vi "Escribir_Arreglo.vi"() -> ()   [LabVIEW 2016]
panel:
  in  "Stop Button":bool
  out "element":i32
  in  "disabled index (col)":i32
  in  "index (row)":i32
  out "Array":i32[][](array[numeric])
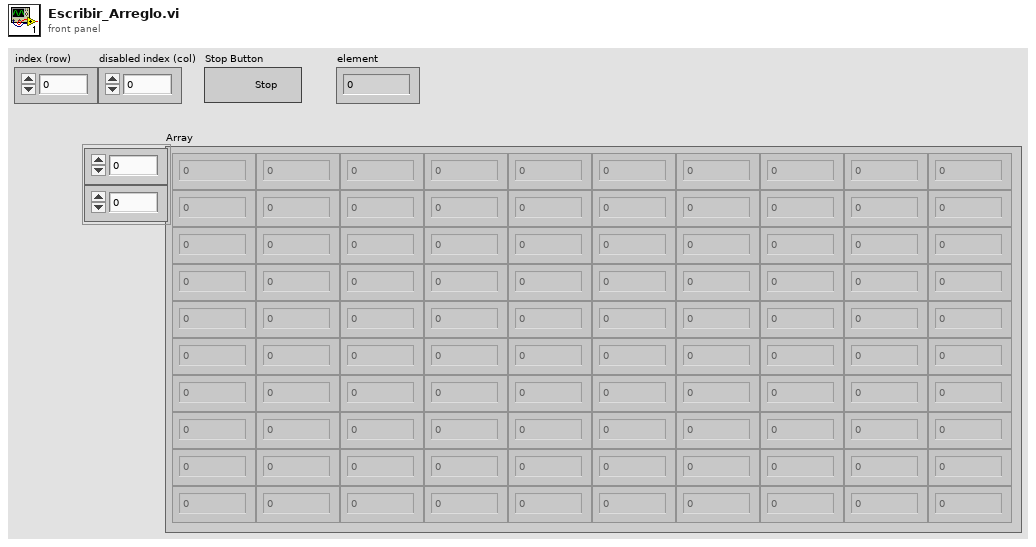
[diagram p1: front panel]
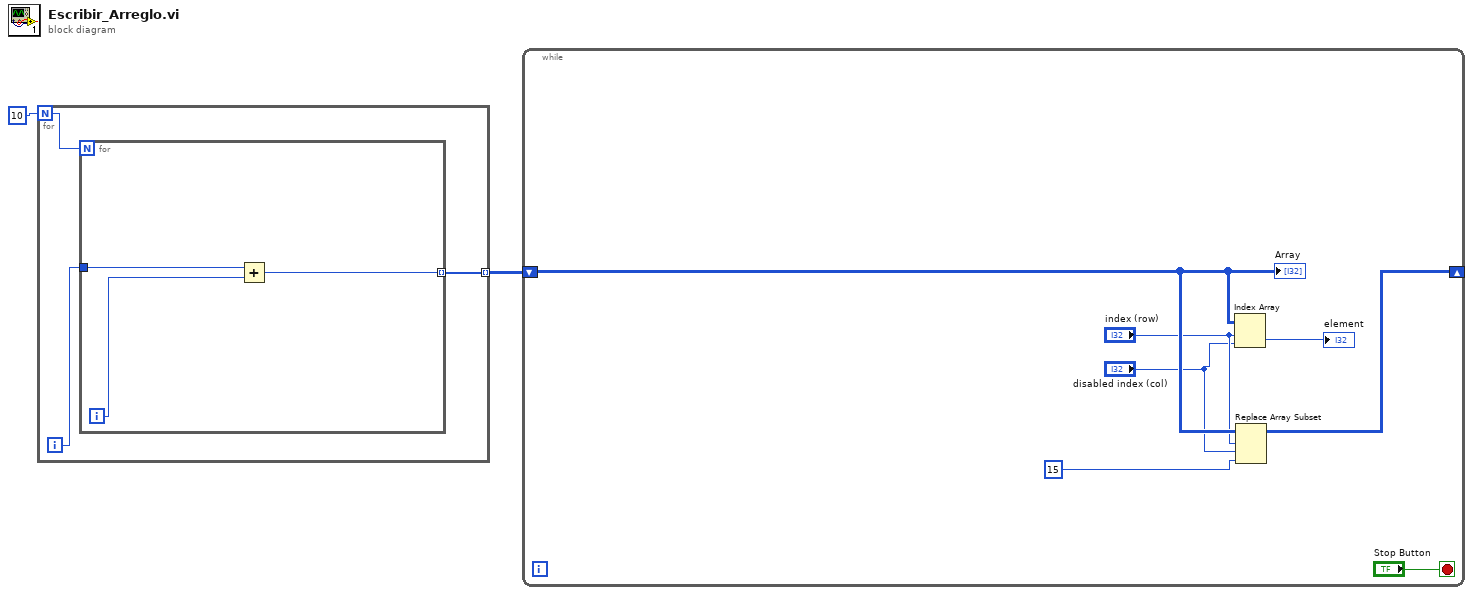
[diagram p0: block diagram]
diagram:
  n1 = for {
    N: 10 -> [w3]
    tunnel: [w4] -> w1 mode=indexing
    i -> [w5]
    n2 = for {
      N: w3 -> [_]
      tunnel: w5 -> [w7]
      tunnel: [w6] -> w4 mode=indexing
      i -> [w8]
      n3 = Add(x=w7, y=w8) -> (x+y=w6:i32)
    }
  }
  n4 = while {
    shift-right: [w9] -> _
    shift-left: w1 -> [w13]
    stop <- "Stop Button" stop-if-true
    n5 = Index Array(array=w13, index (row)="index (row)", index (col)="disabled index (col)") -> (element=→"element":i32)
    n6 = Replace Array Subset(array=w13, new element=15, index (row)="index (row)", index (col)="disabled index (col)") -> (w9:i32[][])
    "Array" <- w13
  }
